vi "Acceleration-Operation_Test.vi"() -> ()   [LabVIEW 2019]
uses:
  <vilib>/Platform/TimedLoop/XDataNode/timing_clust.ctl
  <vilib>/Platform/TimedLoop/XDataNode/nitl_modes.ctl
  <vilib>/Platform/TimedLoop/XDataNode/wakeup.ctl
  <vilib>/platform/TimedLoop/XDataNode/XDataNode.xnode
  <vilib>/Platform/TimedLoop/XDataNode/XDNodeRunTimeDep.lvlib
panel:
  in  "Reset":bool
  out "三角形?":bool
  in  "Stop":bool
  out "Waveform Chart":dbl(graph)
  in  "計算設置":cluster{"總位移量":dbl, "最高速":dbl, "加速度":dbl}={"總位移量"=0.0, "最高速"=75.0, "加速度"=65.0}
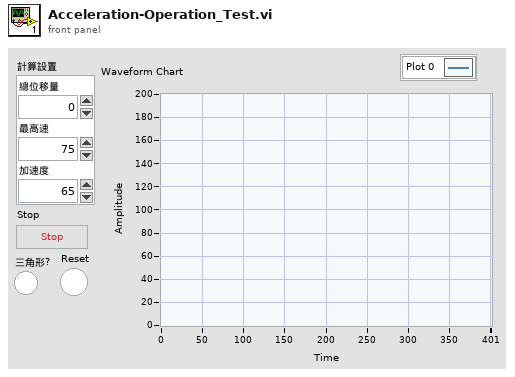
[diagram p1: front panel]
types:
  T1 = typedef "XDNodeRunTimeDep.lvlib/timing_clust.ctl" = cluster{"Expected End [f-1]":u64, "Actual End [f-1]":u64, "Finished Late? [f-1]":bool, "Expected End [i-1]":u64, "Actual End [i-1]":u64, "Finished Late? [i-1]":bool, "Expected Start [i]":u64, "Actual Start [i]":u64, "Expected Start [f]":u64, "Actual Start [f]":u64, "Source Name":string, "Structure Name":string, "Period":i64, "Deadline":i64, "Offset":i64, "Start":i64, "Priority":i32, "Timeout":i32, "Mode":T2, "Wakeup Reason":T3, "Error":errorcluster, "Source Type":string, "Secondary Source Type":string, "Global End Time":u64, "Global Start Time":u64, "Frame Duration":u64, "Iteration Duration":u64, "Assigned CPU":i32, "I/O Scan Engine Mode":u32}
  T2 = typedef "XDNodeRunTimeDep.lvlib/nitl_modes.ctl" = enum32{"No Change", "Process missed periods, maintain original phase", "Discard missed periods, maintain original phase", "Process missed periods, ignore original phase", "Discard missed periods, ignore original phase"}
  T3 = typedef "XDNodeRunTimeDep.lvlib/wakeup.ctl" = enum32{"Normal", "Aborted", "Asynchronous wakeup", "Timing source error", "Timed loop error", "Timeout"}
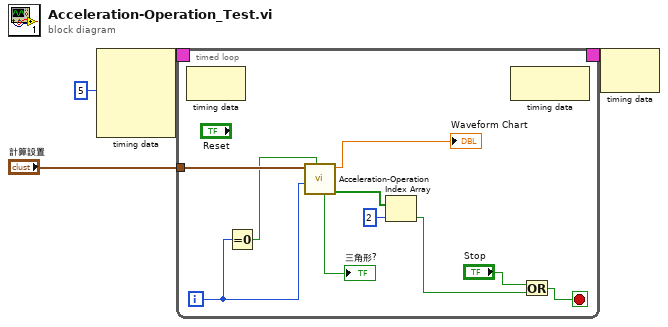
[diagram p0: block diagram]
diagram:
  n1 = node-c288(i64 5 ("Period")) -> (w4:T1)  [unwired: 3 in]
  n2 = timed-loop {
    timing: w4 -> [_]
    timing-out: [_] -> w3
    tunnel: "計算設置" -> [w14]
    i -> [w6]
    stop <- w11 stop-if-true
    n3 = node-c288() -> ()  [unwired: 1 in, 1 out]
    n4 = Equal To 0?(x=w6) -> (x = 0?=w5:bool)
    n5 = call "Acceleration-Operation.vi"("Reset"=w5, "迴圈( I )"=w6, "計算設置"=w14) -> ("完成?"=w13:bool[], "速度"=→"Waveform Chart":dbl, "三角形?"=→"三角形?":bool)  [unwired: 6 in]
    n6 = Index Array(array=w13, index=2) -> (element=w10:bool)
    n7 = node-c288() -> ()  [unwired: 1 in, 1 out]
    n8 = Or(x="Stop", y=w10) -> (x .or. y?=w11:bool)
  }
  n9 = node-c288(w3) -> ()  [unwired: 1 out]
